vi "Write VI Refnum.vi"(8 "Error In":errorcluster, 10 "VI Refnum":refnum<vi>, 11 "Model in":refnum<class "Model.lvclass">) -> (0 "Error Out":errorcluster, 3 "Model out":refnum<class "Model.lvclass">)   [LabVIEW 2021, in "Model.lvclass"]
uses:
  Model.lvclass
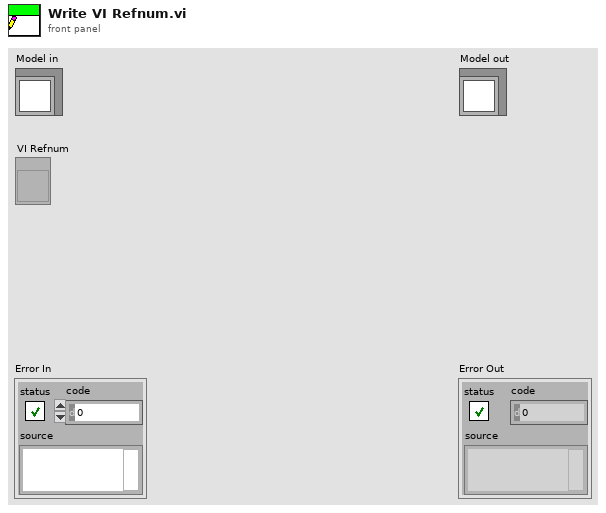
[diagram p1: front panel]
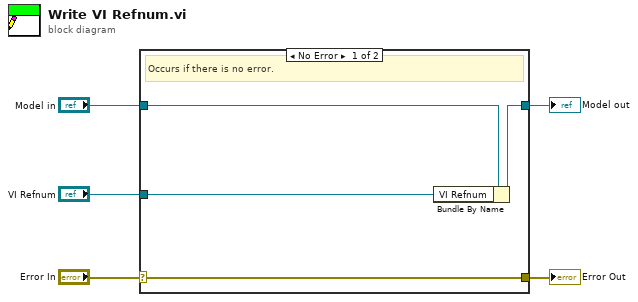
[diagram p0: block diagram]
diagram:
  n1 = case shown="No Error" "Error In" {
    selector: "Error In" -> [w9 w10]
    tunnel: [w9 w10] -> w4
    tunnel: [w7 w11] -> w2
    tunnel: "Model in" -> [w8 w11]
    tunnel: "VI Refnum" -> [w6 _]
    frame No Error {
      # "Occurs if there is no error."
      n2 = Bundle By Name(cluster=w8, "VI Refnum"=w6) -> (w7:refnum<class "Model.lvclass">)
    }
    frame Error {
      # "Occurs if there is any error."
    }
  }
  "Error Out" <- w4
  "Model out" <- w2
